vi "Extrahieren.vi"(9 "Cal Gase":u16[](array[numeric]), 11 "Messbereiche":u16[](array[numeric])) -> (1 "Cal Gase":u16[](array[numeric]), 3 "Messbereiche":u16[](array[numeric]))   [LabVIEW 2020, in "CalGas Aufschaltung.lvlib"]
uses:
  CalGas Aufschaltung.lvlib
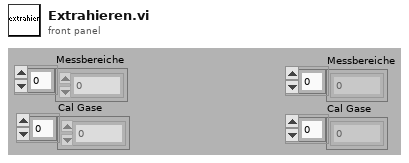
[diagram p1: front panel]
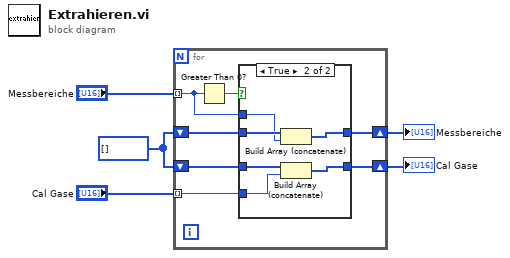
[diagram p0: block diagram]
diagram:
  w5 = u16[] []
  n1 = for {
    shift-right: [w10] -> w1
    shift-left: w5 -> [w11]
    tunnel: "Messbereiche" -> [w7] mode=indexing
    tunnel: "Cal Gase" -> [w9] mode=indexing
    shift-right: [w6] -> w2
    shift-left: w5 -> [w8]
    n2 = Greater Than 0?(x=w7) -> (x > 0?=w12:bool)
    n3 = case shown="True" w12 {
      tunnel: w11 -> [w14 w20]
      tunnel: [w14 w19] -> w10
      tunnel: w9 -> [_ w18]
      tunnel: w8 -> [w13 w16]
      tunnel: w7 -> [_ w15]
      tunnel: [w13 w17] -> w6
      frame False {
      }
      frame True {
        n4 = Build Array (concatenate)(w16, w15) -> (w17:u16[])
        n5 = Build Array (concatenate)(w20, w18) -> (w19:u16[])
      }
    }
  }
  "Messbereiche" <- w2
  "Cal Gase" <- w1
